vi "EventBuilder.init.vi"(0 "i ref in":refnum<vi>, 1 "header":T1, 2 "DAQ objects":string[](array[string]), 3 "ms timeout (10000)":i32=10000, 5 "error in (no error)":errorcluster) -> (14 "i ref out":refnum<vi>, 17 "timed out":bool, 19 "error out":errorcluster)   [LabVIEW 2014, in "EventBuilder.lvlib"]
doc: "Sets a \"header\" of the data and the names of the DAQ devices and publishes a DIM service \"EVENTBUILDERNAME_dataDesciption\"."
uses:
  EventBuilder.lvlib
  CS_Core/CSSystem/CoreDefs/CoreDefs.rawDataType.ctl
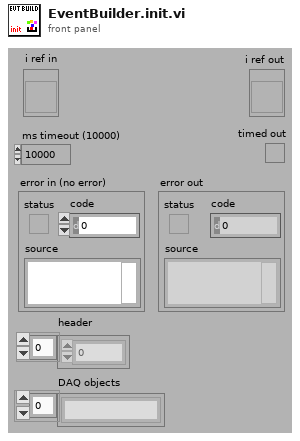
[diagram p1: front panel]
types:
  T1 = typedef "CoreDefs.rawDataType.ctl" = i8[]
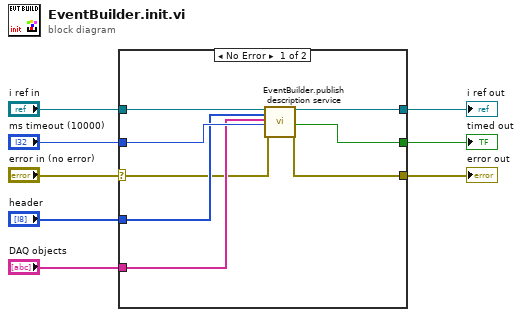
[diagram p0: block diagram]
diagram:
  n1 = case shown="No Error" "error in (no error)" {
    selector: "error in (no error)" -> [w10 w17]
    tunnel: "i ref in" -> [w16 w18]
    tunnel: "ms timeout (10000)" -> [w15 _]
    tunnel: [w12 _] -> w6
    tunnel: "DAQ objects" -> [w13 _]
    tunnel: "header" -> [w14 _]
    tunnel: [w9 w17] -> w3
    tunnel: [w11 w18] -> w2
    frame No Error {
      n2 = call "EventBuilder.publish description service.vi"("i ref in"=w16, "myHeaderData"=w14, "DAQDevices"=w13, "ms timeout (10000)"=w15, "error in (no error)"=w10) -> ("i ref out"=w11:refnum<vi>, "timed out"=w12:bool, "error out"=w9:errorcluster)  [unwired: 12 in]
    }
    frame Error {
    }
  }
  "error out" <- w3
  "i ref out" <- w2
  "timed out" <- w6
